vi "Convert_R-T.vi"(1 "Resistance R":dbl) -> (0 "Temperature C":dbl)   [LabVIEW 2022 SP3]
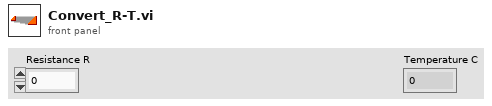
[diagram p1: front panel]
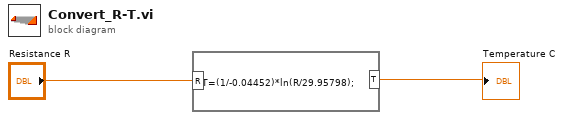
[diagram p0: block diagram]
diagram:
  n1 = formula code="T=(1/-0.04452)*ln(R/29.95798);"("R"="Resistance R") -> ("T"=→"Temperature C":dbl)
